vi "梦幻城堡C1~3界面.vi"() -> ()   [LabVIEW 2016, in "环境动力监测库.lvlib" / "UPS库.lvlib"]
panel:
  out "x+1":u32
  in  "解除告警":bool
  out "状态":T1
  out "通信":bool=TRUE
  out "串口":string
  in  "查看型号":bool
  out "关机倒计时":i32
  out "关闭中":bool
  out "UPS状态":T2
  in  "关机":bool
  in  "重开串口":bool
  # "输入电压"
  # "V"
  # "V"
  # "输入故障电压"
  # "输出电压"
  # "V"
  # "输出电流"
  # "A"
  # "输入频率"
  # "Hz"
  # "电池电压"
  # "V"
  # "UPS温度"
  # "℃"
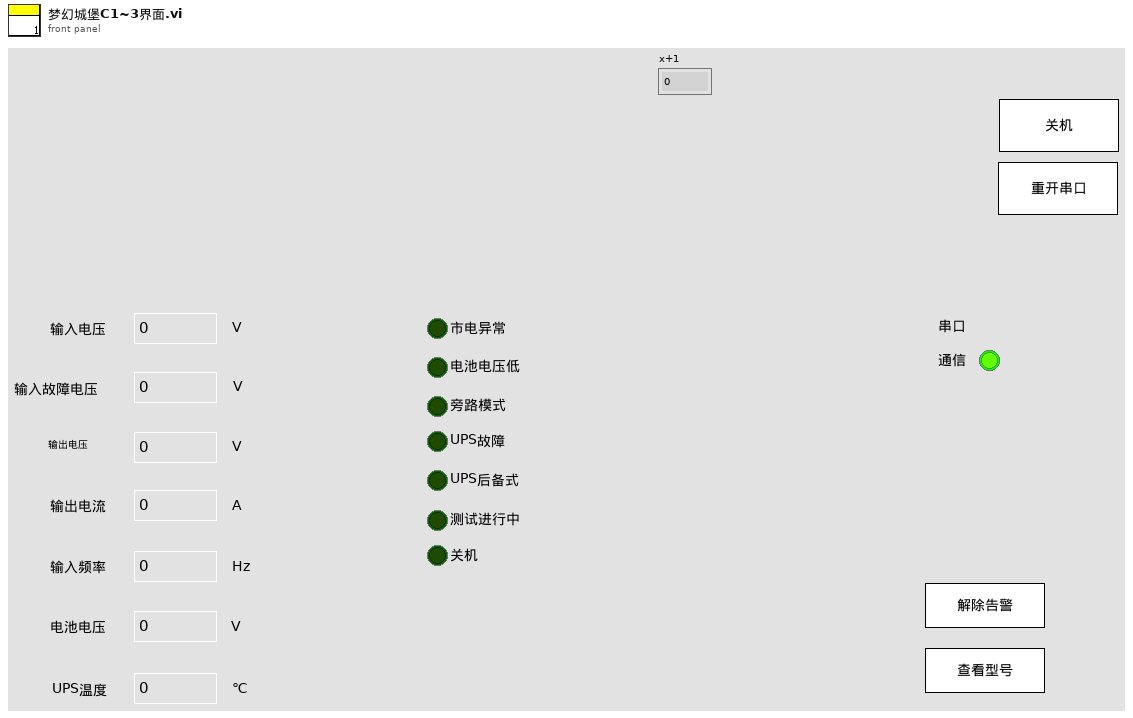
[diagram p1: front panel]
types:
  T1 = cluster{"I/P voltage":dbl, "I/P fault voltage":dbl, "O/P voltage":dbl, "O/P load %":dbl, "I/P frequency HZ":dbl, "Battery voltage":dbl, "Temperature":dbl}
  T2 = cluster{"市电异常":bool, "电池电压低":bool, "旁路模式":bool, "UPS故障":bool, "UPS后备式":bool, "测试进行中":bool, "关机":bool, "保留":bool}
  T3 = cluster{"枚举":enum16{"open", "read", "write", "close"}, "写入缓冲区":string}
  T4 = enum32{"Bad", "Idle", "Run top level", "Running"}
  T5 = cluster{"漏水监测输出":cluster{"漏水监测告警":bool, "告警内容":string}, "门禁监测输出":cluster{"门禁监测告警":bool, "告警内容":string}, "门禁监测输出2":cluster{"门禁监测告警":bool, "告警内容":string}, "温湿度监测输出":cluster{"温湿度监测告警":bool, "告警内容":string}, "烟雾监测输出":cluster{"烟雾监测告警":bool, "告警内容":string}, "空调监测输出":cluster{"空调监测告警":bool, "告警内容":string}, "自动重合闸输出":cluster{"自动重合闸告警":bool, "告警内容":string}, "红外入侵输出":cluster{"红外入侵告警":bool, "告警内容":string}, "振动输出":cluster{"振动告警":bool, "告警内容":string}, "UPS输出":cluster{"UPS告警":bool, "告警内容":string}, "蓄电池输出":cluster{"蓄电池告警":bool, "告警内容":string}, "蓄电池输出2":cluster{"蓄电池告警":bool, "告警内容":string}, "GPS输出":cluster{"定位告警":bool, "告警内容":string}, "北斗输出":cluster{"定位告警":bool, "告警内容":string}, "气象输出":cluster{"气象告警":bool, "告警内容":string}, "废液输出":cluster{"废液告警":bool, "告警内容":string}, "废液输出2":cluster{"废液告警":bool, "告警内容":string}}
  T6 = cluster{"VISA resource name":refnum<visa-resource-name>, "Serial Config":cluster{"baud rate (9600)":u32, "stop bits (10: 1 bit)":u16, "parity (0:none)":enum16{"None", "Odd", "Even", "Mark", "Space"}, "data bits (8)":u16, "timeout (10sec)":u32}, "型号选择":enum16{"山特UPSC1~3", "山特UPSC6~20", "华为UPS2000-G-(1-3KVA)"}, "HW-UPS-2000 MB session":refnum<class "MB_Master.lvclass">, "连接方式":enum16{"串口", "TCP"}, "IP":string, "Port":string}
  T7 = cluster{"I/P voltage":dbl, "I/P fault voltage":dbl, "O/P voltage":dbl, "O/P load %":dbl, "I/P frequency HZ":dbl, "Battery voltage":dbl, "Temperature":dbl, "U":string}
  T8 = cluster{"市电":cluster{"状态":bool, "电压:":u16, "电流：":dbl, "详情  ":bool}, "UPS":cluster{"状态":bool, "输入电压:":sgl, "输出电压:":sgl, "电池电量:":u8, "电量":u16, "详情  ":bool}, "蓄电池12V":cluster{"状态":bool, "电压:":sgl, "电流:":sgl, "电池电量:":u8, "电量":u16, "详情  ":bool, "充电":bool, "负载":bool}, "蓄电池24V":cluster{"状态":bool, "电压:":sgl, "电流:":sgl, "电池电量:":u8, "电量":u16, "详情  ":bool, "充电":bool, "负载":bool}}
  T9 = cluster{"[0]":bool, "[1]":bool, "[2]":bool, "[3]":bool, "[4]":bool, "[5]":bool, "[6]":bool, "[7]":bool}
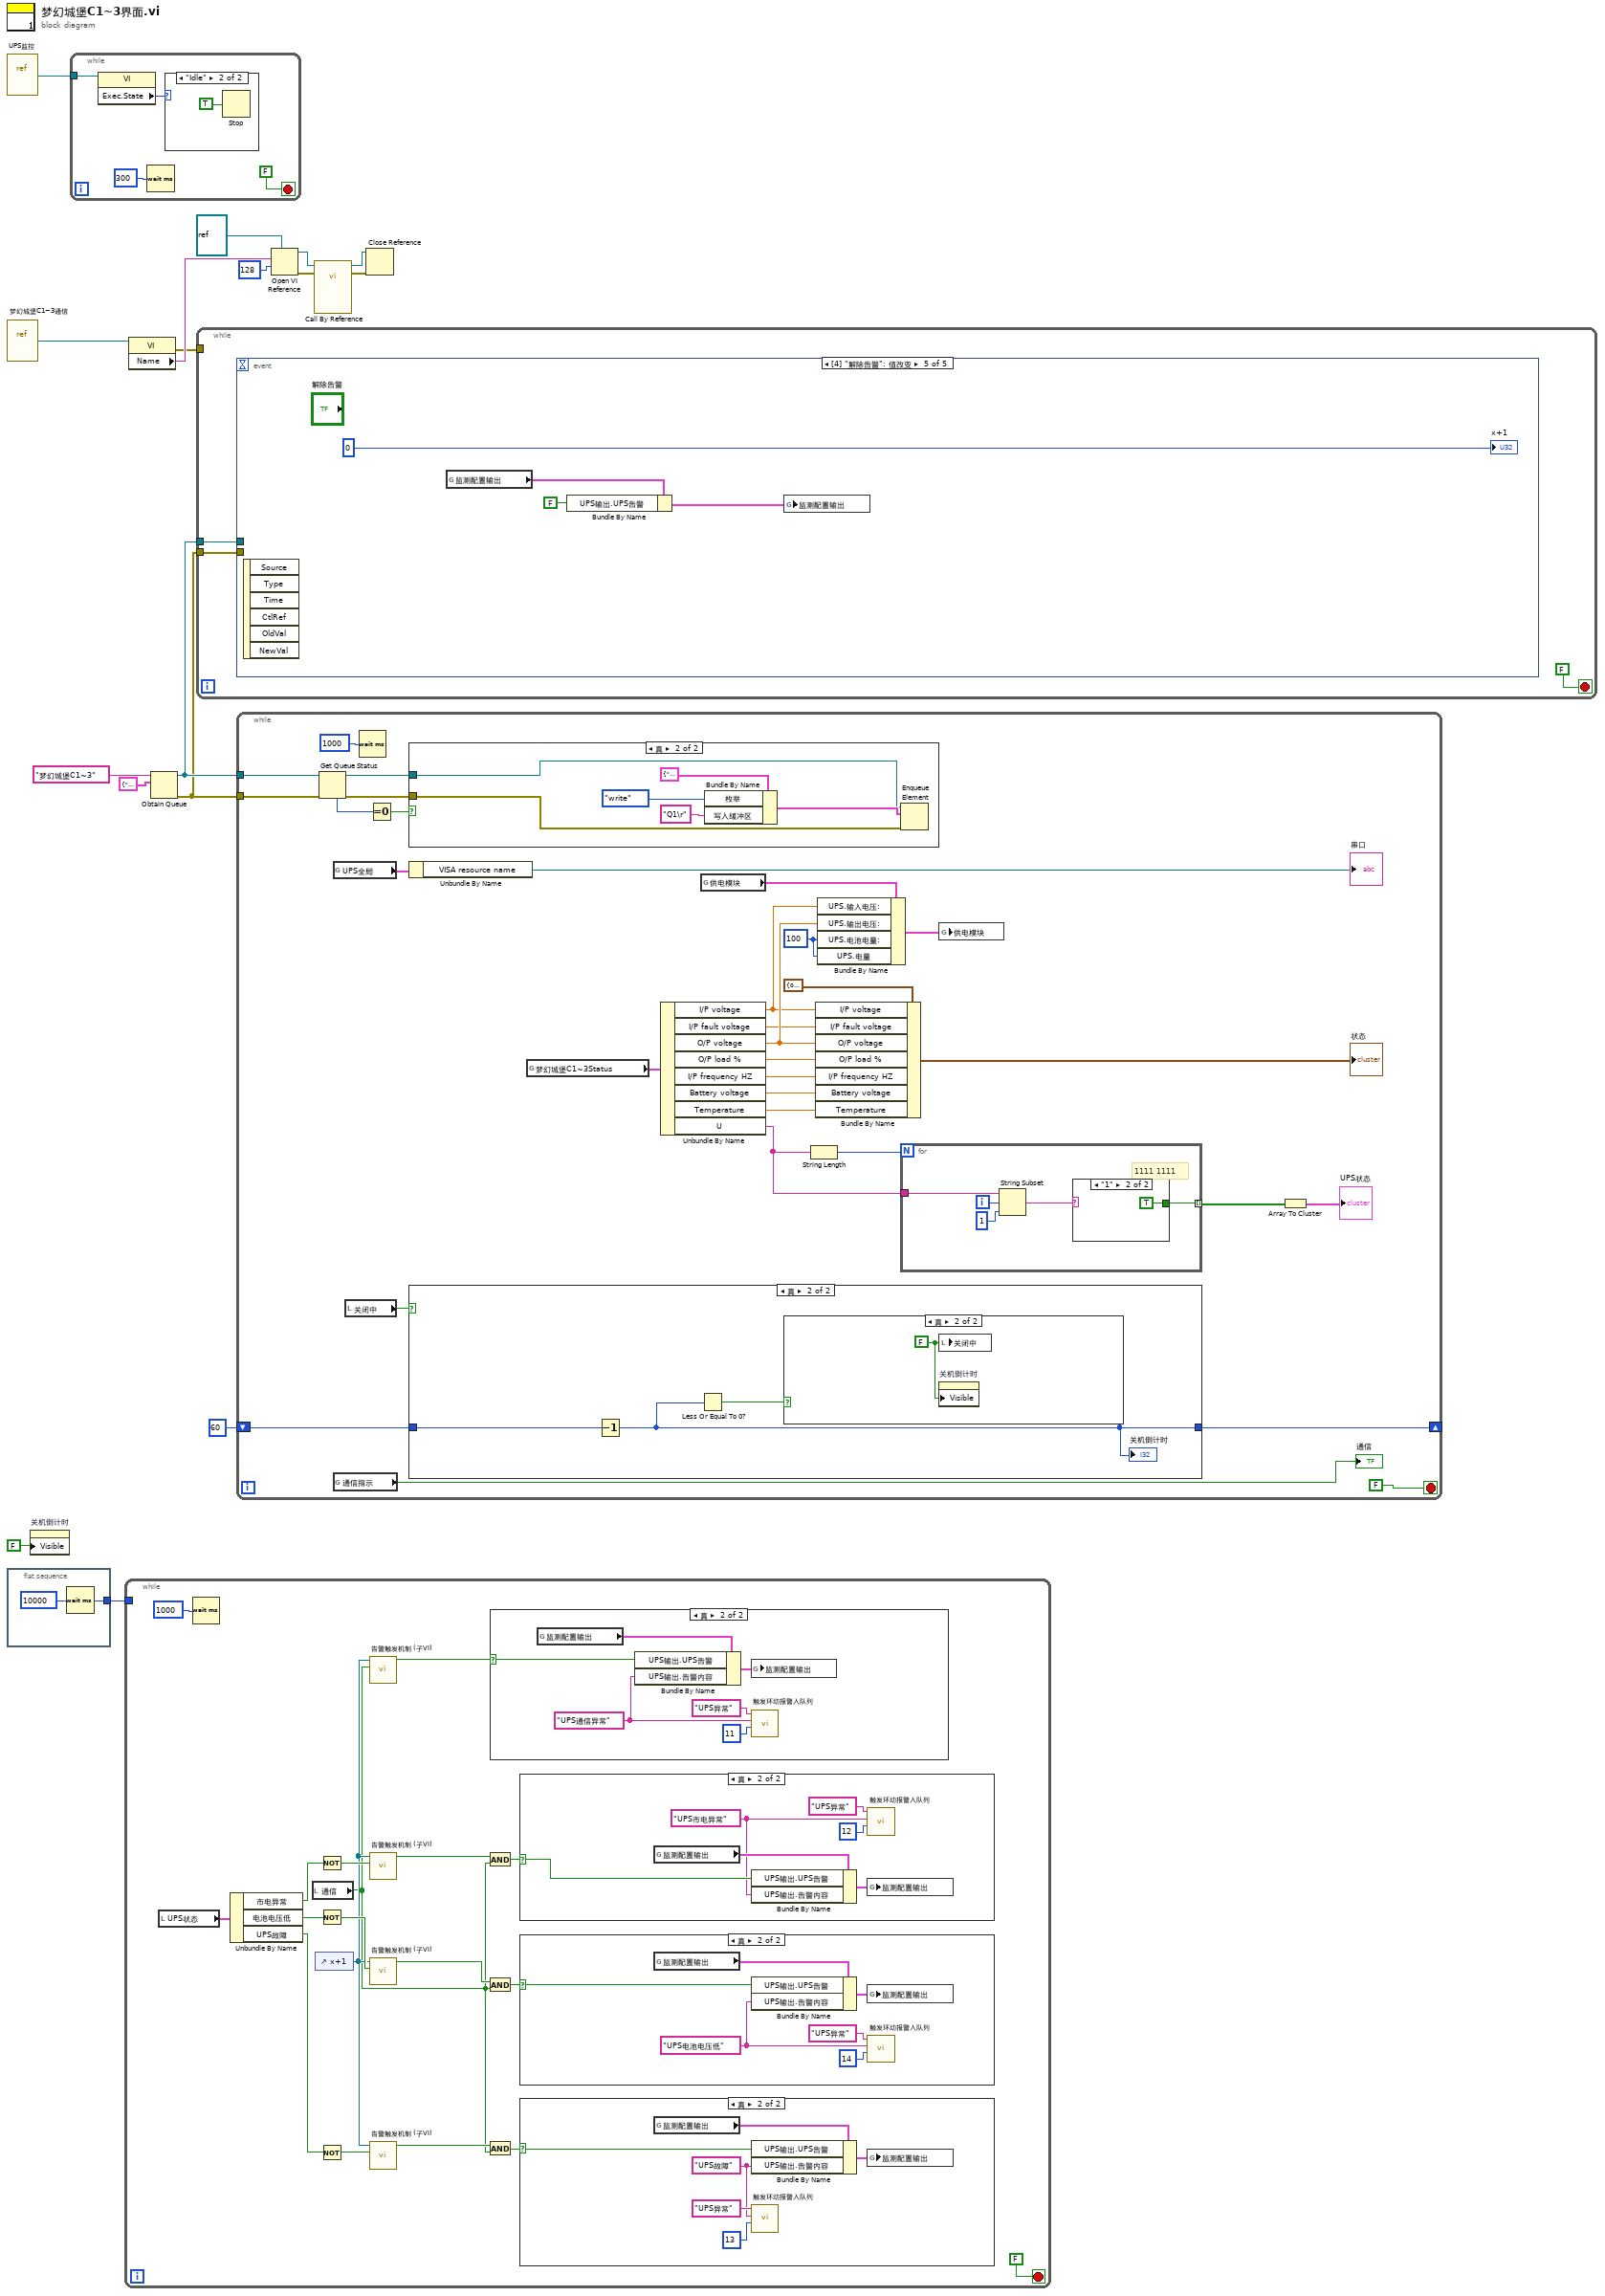
[diagram p0: block diagram]
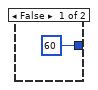
[diagram p8: hidden frame]
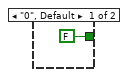
[diagram p10: hidden frame]
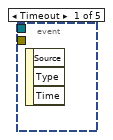
[diagram p11: hidden frame]
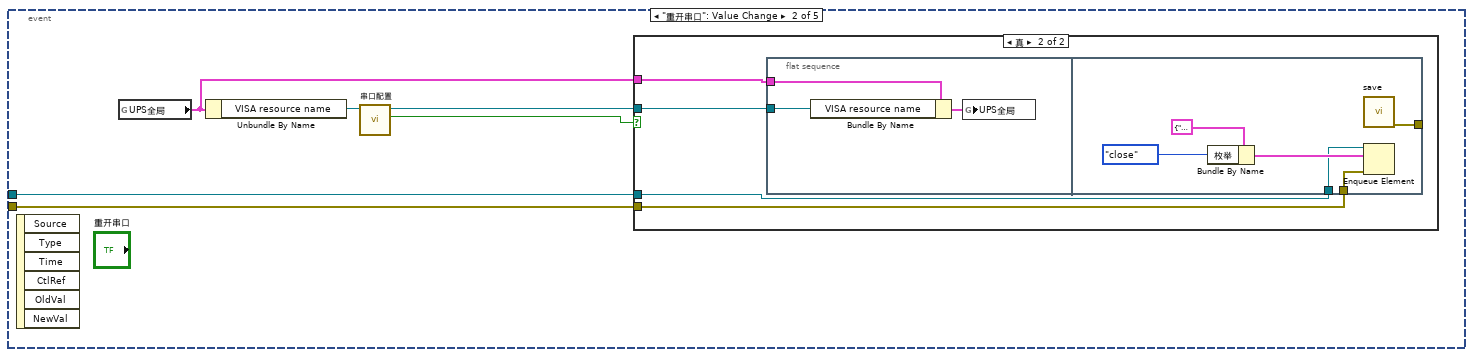
[diagram p12: hidden frame]
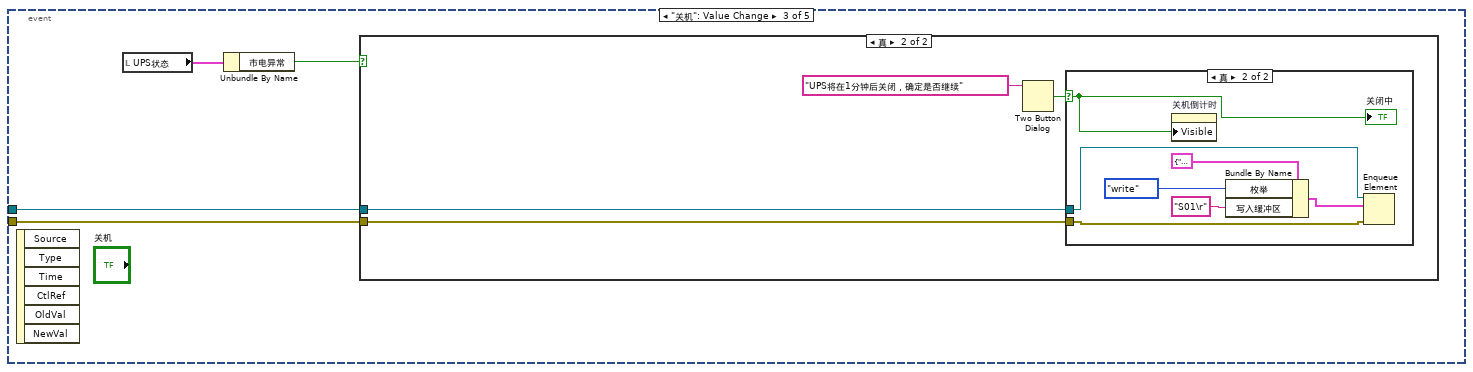
[diagram p14: hidden frame]
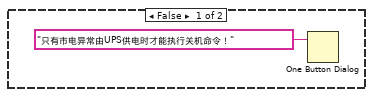
[diagram p15: hidden frame]
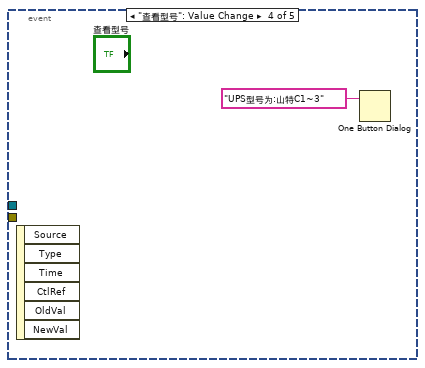
[diagram p17: hidden frame]
diagram:
  n1 = vi-ref "UPS监控.vi"() -> (w2:refnum<vi>)
  n2 = vi-ref "梦幻城堡C1~3通信.vi"() -> (w10:refnum<vi>)
  n3 = flat-sequence {
    tunnel: [w18] -> w1
    frame #0 {
      n4 = Wait (ms)(milliseconds to wait=u32 10000 ("等待时间（毫秒）")) -> (millisecond timer value=w18:u32)
    }
  }
  n5 = property on="关机倒计时" class="DigNum (严格)"("Visible"=FALSE ("可见")) -> ()  [unwired: 2 in, 2 out]
  n6 = while {
    tunnel: w2 -> [w23]
    stop <- FALSE stop-if-true
    n7 = property class="VI"(reference=w23) -> ("Exec.State"=w22:T4)  [unwired: 1 in, 2 out]
    n8 = Wait (ms)(milliseconds to wait=u32 300 ("等待时间（毫秒）")) -> ()  [unwired: 1 out]
    n9 = case shown="\"Idle\"" w22 {
      frame "Bad", Default {
      }
      frame "Idle" {
        n10 = Stop(stop? (T)=TRUE ("停止？(T)")) -> ()
      }
    }
  }
  n11 = while {
    tunnel: w1 -> [_]
    stop <- FALSE stop-if-true
    n12 = local read "UPS状态"() -> (w40:T2)
    n13 = Wait (ms)(milliseconds to wait=u32 1000 ("等待时间（毫秒）")) -> ()  [unwired: 1 out]
    n14 = Unbundle By Name(w40) -> ("市电异常"=w34:bool, "电池电压低"=w31:bool, "UPS故障"=w37:bool)
    n15 = local read "通信"() -> (w25:bool)
    n16 = control-ref of="x+1"() -> (w29:refnum<vi>)
    n17 = Not(x=w34) -> (.not. x?=w35:bool)
    n18 = Not(x=w31) -> (.not. x?=w32:bool)
    n19 = Not(x=w37) -> (.not. x?=w38:bool)
    n20 = call "告警触发机制 (子VI).vi"("状态输出"=w25, "Digital输入"=w29) -> ("触发告警"=w39:bool)  [unwired: 8 in, 1 out]
    n21 = call "告警触发机制 (子VI).vi"("状态输出"=w35, "Digital输入"=w29) -> ("触发告警"=w33:bool)  [unwired: 8 in, 1 out]
    n22 = call "告警触发机制 (子VI).vi"("状态输出"=w32, "Digital输入"=w29) -> ("触发告警"=w30:bool)  [unwired: 8 in, 1 out]
    n23 = call "告警触发机制 (子VI).vi"("状态输出"=w38, "Digital输入"=w29) -> ("触发告警"=w36:bool)  [unwired: 8 in, 1 out]
    n24 = And(x=w33, y=w25) -> (x .and. y?=w28:bool)
    n25 = And(x=w30, y=w25) -> (x .and. y?=w27:bool)
    n26 = And(x=w36, y=w25) -> (x .and. y?=w26:bool)
    n27 = case shown="真" w39 {
      selector: w39 -> [_ w48]
      frame False {
      }
      frame True {
        w44 = "UPS通信异常" ("报警内容")
        n28 = global read "内部交互全局变量.vi" "监测配置输出"() -> (w46:T5)
        n29 = Bundle By Name(cluster=w46, "UPS输出.UPS告警"=w48, "UPS输出.告警内容"=w44) -> (w47:T5)
        n30 = global write "内部交互全局变量.vi" "监测配置输出"(w47) -> ()
        n31 = call "触发环动报警入队列.vi"("code"=11, "告警详情"=w44, "告警信息"="UPS异常" ("设备")) -> ()  [unwired: 9 in]
      }
    }
    n32 = case shown="真" w28 {
      selector: w28 -> [_ w66]
      frame False {
      }
      frame True {
        w63 = "UPS市电异常" ("报警内容")
        n33 = global read "内部交互全局变量.vi" "监测配置输出"() -> (w65:T5)
        n34 = Bundle By Name(cluster=w65, "UPS输出.UPS告警"=w66, "UPS输出.告警内容"=w63) -> (w64:T5)
        n35 = call "触发环动报警入队列.vi"("code"=12, "告警详情"=w63, "告警信息"="UPS异常" ("设备")) -> ()  [unwired: 9 in]
        n36 = global write "内部交互全局变量.vi" "监测配置输出"(w64) -> ()
      }
    }
    n37 = case shown="真" w27 {
      selector: w27 -> [_ w60]
      frame False {
      }
      frame True {
        w56 = "UPS电池电压低" ("报警内容")
        n38 = global read "内部交互全局变量.vi" "监测配置输出"() -> (w59:T5)
        n39 = Bundle By Name(cluster=w59, "UPS输出.UPS告警"=w60, "UPS输出.告警内容"=w56) -> (w58:T5)
        n40 = global write "内部交互全局变量.vi" "监测配置输出"(w58) -> ()
        n41 = call "触发环动报警入队列.vi"("code"=14, "告警详情"=w56, "告警信息"="UPS异常" ("设备")) -> ()  [unwired: 9 in]
      }
    }
    n42 = case shown="真" w26 {
      selector: w26 -> [_ w54]
      frame False {
      }
      frame True {
        w50 = "UPS故障" ("报警内容")
        n43 = global read "内部交互全局变量.vi" "监测配置输出"() -> (w53:T5)
        n44 = Bundle By Name(cluster=w53, "UPS输出.UPS告警"=w54, "UPS输出.告警内容"=w50) -> (w52:T5)
        n45 = call "触发环动报警入队列.vi"("code"=13, "告警详情"=w50, "告警信息"="UPS异常" ("设备")) -> ()  [unwired: 9 in]
        n46 = global write "内部交互全局变量.vi" "监测配置输出"(w52) -> ()
      }
    }
  }
  n47 = property class="VI"(reference=w10) -> (error out=w4:errorcluster, "Name"=w11:string)  [unwired: 1 in, 1 out]
  n48 = Obtain Queue(name (unnamed)="梦幻城堡C1~3" ("名称（未命名）"), element data type=T3 {"枚举"=enum."open", "写入缓冲区"=""}) -> (queue out=w7:refnum<queue>, error out=w6:errorcluster)  [unwired: 3 in, 1 out]
  n49 = while {
    tunnel: w6 -> [w68]
    tunnel: w7 -> [w67]
    tunnel: w4 -> [_]
    stop <- FALSE stop-if-true
    n50 = event shown="[4] \"解除告警\": 值改变" {
      selector: _ -> [_ _ _ _ _]
      dyn-events: _ -> [_ _ _ _ _]
      timeout: _ -> [_ _ _ _ _]
      tunnel: w68 -> [_ w72 w91 _ _]
      tunnel: w67 -> [_ w73 w92 _ _]
      event Timeout {
        n51 = event-data() -> ()  [unwired: 1 in, 3 out]
      }
      event "重开串口": Value Change {
        n52 = event-data() -> ()  [unwired: 1 in, 6 out]
        n53 = global read "断电保存全局变量.vi" "UPS全局"() -> (w70:T6)
        n54 = Unbundle By Name(w70) -> ("VISA resource name"=w71:refnum<visa-resource-name>)
        n55 = call "串口配置.vi"("请选择串口:"=w71) -> ("确认 2"=w75:bool, "请选择串口: 2"=w74:refnum<visa-resource-name>)  [unwired: 9 in]
        n56 = case shown="真" w75 {
          tunnel: w74 -> [_ w79]
          tunnel: w73 -> [_ w78]
          tunnel: w72 -> [_ w77]
          tunnel: w70 -> [_ w76]
          frame False {
          }
          frame True {
            n57 = flat-sequence {
              tunnel: w79 -> [w80]
              tunnel: w76 -> [w82]
              tunnel: w78 -> [w85]
              tunnel: w77 -> [w84]
              tunnel: [w83] -> _
              frame #0 {
                n58 = Bundle By Name(cluster=w82, "VISA resource name"=w80) -> (w81:T6)
                n59 = global write "断电保存全局变量.vi" "UPS全局"(w81) -> ()
              }
              frame #1 {
                n60 = Bundle By Name(cluster=T3 {"枚举"=enum."open", "写入缓冲区"=""}, "枚举"=enum16{"open", "read", "write", "close"}."close") -> (w88:T3)
                n61 = call "save.vi"() -> ("error out"=w83:errorcluster)  [unwired: 11 in]
                n62 = Enqueue Element(queue=w85, element=w88, error in (no error)=w84) -> ()  [unwired: 1 in, 3 out]
              }
            }
          }
        }
      }
      event "关机": Value Change {
        n63 = event-data() -> ()  [unwired: 1 in, 6 out]
        n64 = local read "UPS状态"() -> (w90:T2)
        n65 = Unbundle By Name(w90) -> ("市电异常"=w89:bool)
        n66 = case shown="真" w89 {
          tunnel: w92 -> [_ w97]
          tunnel: w91 -> [_ w96]
          frame False {
            n67 = One Button Dialog(message="只有市电异常由UPS供电时才能执行关机命令！" ("消息")) -> ()  [unwired: 1 in, 1 out]
          }
          frame True {
            n68 = Two Button Dialog(message="UPS将在1分钟后关闭，确定是否继续" ("消息")) -> (T button?=w94:bool)  [unwired: 2 in]
            n69 = case shown="真" w94 {
              selector: w94 -> [_ w98]
              tunnel: w97 -> [_ w101]
              tunnel: w96 -> [_ w100]
              frame False {
              }
              frame True {
                n70 = property on="关机倒计时" class="DigNum (严格)"("Visible"=w98) -> ()  [unwired: 2 in, 2 out]
                n71 = Bundle By Name(cluster=T3 {"枚举"=enum."open", "写入缓冲区"=""}, "枚举"=enum16{"open", "read", "write", "close"}."write", "写入缓冲区"="S01\r") -> (w102:T3)
                n72 = Enqueue Element(queue=w101, element=w102, error in (no error)=w100) -> ()  [unwired: 1 in, 3 out]
                "关闭中" <- w98
              }
            }
          }
        }
      }
      event "查看型号": Value Change {
        n73 = event-data() -> ()  [unwired: 1 in, 6 out]
        n74 = One Button Dialog(message="UPS型号为:山特C1~3" ("消息")) -> ()  [unwired: 1 in, 1 out]
      }
      event "解除告警": Value Change {
        n75 = event-data() -> ()  [unwired: 1 in, 6 out]
        n76 = global read "内部交互全局变量.vi" "监测配置输出"() -> (w107:T5)
        n77 = Bundle By Name(cluster=w107, "UPS输出.UPS告警"=FALSE) -> (w106:T5)
        n78 = global write "内部交互全局变量.vi" "监测配置输出"(w106) -> ()
        "x+1" <- u32 0 ("x+1")
      }
    }
  }
  n79 = while {
    tunnel: w7 -> [w130]
    tunnel: w6 -> [w129]
    shift-right: [w132] -> _
    shift-left: 60 -> [w133]
    stop <- FALSE stop-if-true
    w123 = u8 100 ("UPS.电池电量:")
    n80 = Get Queue Status(queue=w130, error in (no error)=w129) -> (queue out=w128:refnum<queue>, error out=w127:errorcluster, # elements in queue=w131:i32)  [unwired: 1 in, 5 out]
    n81 = global read "断电保存全局变量.vi" "UPS全局"() -> (w111:T6)
    n82 = global read "UPS内部交互全局.vi" "通信指示"() -> (→"通信":bool)
    n83 = local read "关闭中"() -> (w134:bool)
    n84 = Wait (ms)(milliseconds to wait=u32 1000 ("等待时间（毫秒）")) -> ()  [unwired: 1 out]
    n85 = Equal To 0?(x=w131) -> (x = 0?=w126:bool)
    n86 = case shown="真" w126 {
      tunnel: w128 -> [_ w142]
      tunnel: w127 -> [_ w141]
      frame False {
      }
      frame True {
        n87 = Bundle By Name(cluster=T3 {"枚举"=enum."open", "写入缓冲区"=""}, "枚举"=enum16{"open", "read", "write", "close"}."write", "写入缓冲区"="Q1\r") -> (w145:T3)
        n88 = Enqueue Element(queue=w142, element=w145, error in (no error)=w141) -> ()  [unwired: 1 in, 3 out]
      }
    }
    n89 = Unbundle By Name(w111) -> ("VISA resource name"=→"串口":refnum<visa-resource-name>)
    n90 = case shown="真" w134 {
      tunnel: w133 -> [_ w150]
      tunnel: [60 w149] -> w132
      frame False {
      }
      frame True {
        n91 = Decrement(x=w150) -> (x-1=w149:i32)
        "关机倒计时" <- w149
        n92 = Less Or Equal To 0?(x=w149) -> (x <= 0?=w148:bool)
        n93 = case shown="真" w148 {
          frame False {
          }
          frame True {
            w151 = FALSE ("关闭中")
            n94 = local write "关闭中"(w151) -> ()
            n95 = property on="关机倒计时" class="DigNum (严格)"("Visible"=w151) -> ()  [unwired: 2 in, 2 out]
          }
        }
      }
    }
    n96 = global read "UPS内部交互全局.vi" "梦幻城堡C1~3Status"() -> (w138:T7)
    n97 = Unbundle By Name(w138) -> ("I/P voltage"=w113:dbl, "I/P fault voltage"=w112:dbl, "O/P voltage"=w114:dbl, "O/P load %"=w115:dbl, "I/P frequency HZ"=w116:dbl, "Battery voltage"=w117:dbl, "Temperature"=w118:dbl, "U"=w135:string)
    n98 = global read "内部交互全局变量.vi" "供电模块"() -> (w125:T8)
    n99 = String Length(string=w135) -> (length=w136:i32)
    n100 = Bundle By Name(cluster=T1 {"I/P voltage"=0.0, "I/P fault voltage"=0.0, "O/P voltage"=0.0, "O/P load %"=0.0, "I/P frequency HZ"=0.0, "Battery voltage"=0.0, "Temperature"=0.0} ("状态"), "I/P voltage"=w113, "I/P fault voltage"=w112, "O/P voltage"=w114, "O/P load %"=w115, "I/P frequency HZ"=w116, "Battery voltage"=w117, "Temperature"=w118) -> (→"状态":T1)
    n101 = Bundle By Name(cluster=w125, "UPS.输入电压:"=w113, "UPS.输出电压:"=w114, "UPS.电池电量:"=w123, "UPS.电量"=w123) -> (w124:T8)
    n102 = for {
      N: w136 -> [_]
      tunnel: w135 -> [w156]
      tunnel: [w152] -> w122 mode=indexing
      i -> [w154]
      # "1111 1111"
      n103 = String Subset(string=w156, offset (0)=w154, length (rest)=1 ("长度（剩余）")) -> (substring=w153:string)
      n104 = case shown="\"1\"" w153 {
        tunnel: [FALSE TRUE] -> w152
        frame "0", Default {
        }
        frame "1" {
        }
      }
    }
    n105 = global write "内部交互全局变量.vi" "供电模块"(w124) -> ()
    n106 = Array To Cluster(array=w122) -> (cluster=→"UPS状态":T9)
  }
  n107 = Open VI Reference(type specifier VI Refnum (for type only)=refnum<vi> refnum, vi path=w11, options=128 ("选项")) -> (vi reference=w13:refnum<vi>, error out=w15:errorcluster)  [unwired: 3 in]
  n108 = call-by-ref "?"(reference=w13, error in=w15) -> (reference out=w17:refnum<vi>, error out=w16:errorcluster)  [unwired: 12 in]
  n109 = Close Reference(reference=w17, error in (no error)=w16) -> ()  [unwired: 1 out]
